vi "accuracy cal.vi"() -> ()   [LabVIEW 2016]
panel:
  out "원소의 인덱스 2":i32
  out "크기 2":i32
  out "x/y":dbl
  out "원소의 인덱스":i32
  out "정렬된 배열":bool[](array[boolean])
  out "추가된 배열":bool[](array[boolean])
  out "크기":i32
  out "배열 5":dbl[](array[numeric])
  out "배열 4":dbl[](array[numeric])
  out "배열 3":dbl[](array[numeric])
  out "배열 2":dbl[](array[numeric])
  out "배열":dbl[](array[numeric])
  in  "1 5":string
  in  "1 4":string
  in  "1 3":string
  in  "1 2":string
  in  "1":string
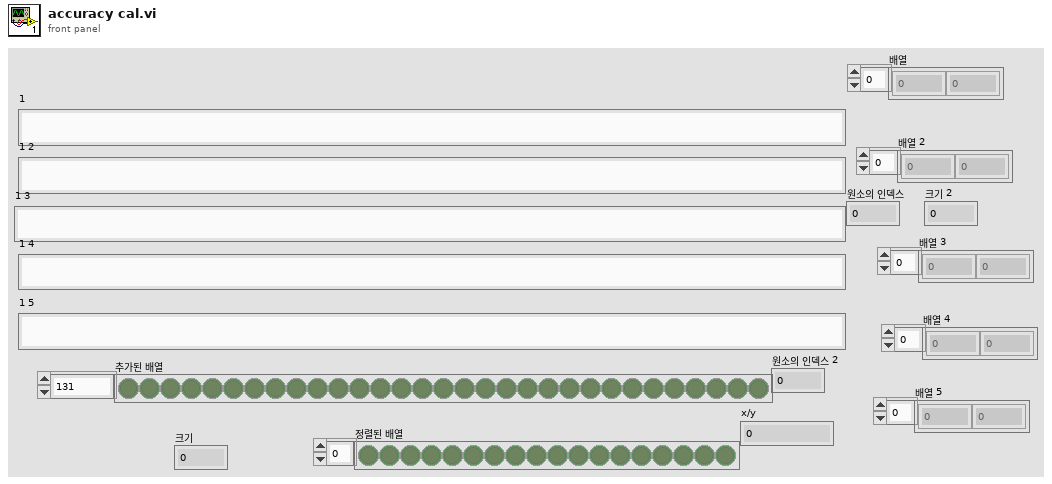
[diagram p1: front panel]
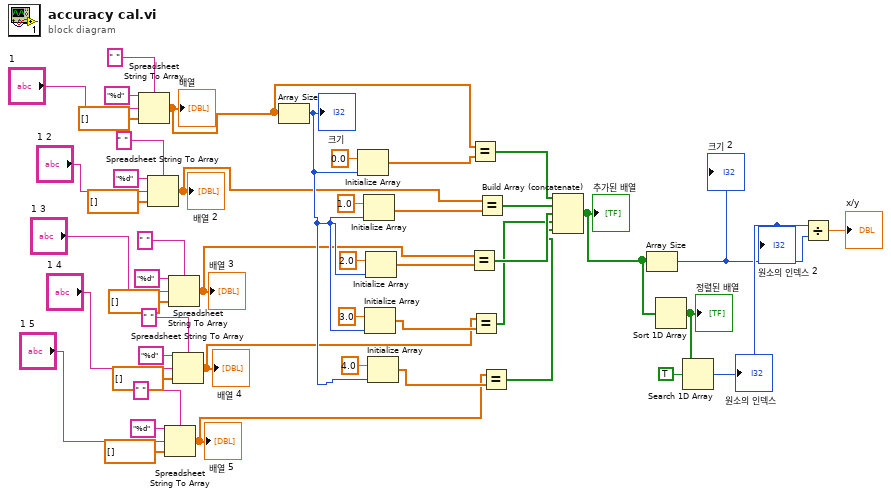
[diagram p0: block diagram]
diagram:
  n1 = Spreadsheet String To Array(delimiter (Tab)=" " ("구분 문자 (탭)"), format string="%d" ("포맷 문자열"), spreadsheet string="1", array type (2D Dbl)=dbl[] [] ("배열 타입(2D Dbl)")) -> (array=w21:dbl[])
  "배열" <- w21
  n2 = Spreadsheet String To Array(delimiter (Tab)=" " ("구분 문자 (탭)"), format string="%d" ("포맷 문자열"), spreadsheet string="1 2", array type (2D Dbl)=dbl[] [] ("배열 타입(2D Dbl)")) -> (array=w19:dbl[])
  "배열 2" <- w19
  n3 = Spreadsheet String To Array(delimiter (Tab)=" " ("구분 문자 (탭)"), format string="%d" ("포맷 문자열"), spreadsheet string="1 5", array type (2D Dbl)=dbl[] [] ("배열 타입(2D Dbl)")) -> (array=w12:dbl[])
  "배열 5" <- w12
  n4 = Spreadsheet String To Array(delimiter (Tab)=" " ("구분 문자 (탭)"), format string="%d" ("포맷 문자열"), spreadsheet string="1 3", array type (2D Dbl)=dbl[] [] ("배열 타입(2D Dbl)")) -> (array=w14:dbl[])
  "배열 3" <- w14
  n5 = Spreadsheet String To Array(delimiter (Tab)=" " ("구분 문자 (탭)"), format string="%d" ("포맷 문자열"), spreadsheet string="1 4", array type (2D Dbl)=dbl[] [] ("배열 타입(2D Dbl)")) -> (array=w13:dbl[])
  "배열 4" <- w13
  n6 = Array Size(array=w21) -> (size(s)=w22:i32)
  "크기" <- w22
  n7 = Initialize Array(0.0 ("원소"), w22) -> (w20:dbl[])
  n8 = Initialize Array(1.0 ("원소"), w22) -> (w18:dbl[])
  n9 = Initialize Array(3.0 ("원소"), w22) -> (w16:dbl[])
  n10 = Initialize Array(2.0 ("원소"), w22) -> (w17:dbl[])
  n11 = Initialize Array(4.0 ("원소"), w22) -> (w15:dbl[])
  n12 = Equal?(x=w14, y=w17) -> (x = y?=w9:bool[])
  n13 = Equal?(x=w21, y=w20) -> (x = y?=w11:bool[])
  n14 = Equal?(x=w13, y=w16) -> (x = y?=w8:bool[])
  n15 = Equal?(x=w19, y=w18) -> (x = y?=w10:bool[])
  n16 = Equal?(x=w12, y=w15) -> (x = y?=w7:bool[])
  n17 = Build Array (concatenate)(w11, w10, w9, w8, w7) -> (w6:bool[])
  "추가된 배열" <- w6
  n18 = Array Size(array=w6) -> (size(s)=w2:i32)
  "크기 2" <- w2
  n19 = Sort 1D Array(array=w6) -> (sorted array=w5:bool[])
  "정렬된 배열" <- w5
  n20 = Search 1D Array(1D array=w5, element=TRUE ("원소")) -> (index of element=w3:i32)  [unwired: 1 in]
  "원소의 인덱스" <- w3
  "원소의 인덱스 2" <- w3
  n21 = Divide(x=w3, y=w2) -> (x/y=→"x/y":dbl)
